vi "test game logic.vi"() -> ()   [LabVIEW 2024]
uses:
  state machine variables.ctl
  state machine states.ctl
  state machine controller.ctl
panel:
  out "Sequence":dbl[](array[numeric])
  in  "Button 4":bool
  in  "Button3":bool
  in  "Button 2":bool
  in  "Button 1":bool
  in  "Round":dbl
  in  "Score":dbl
  in  "stop":bool
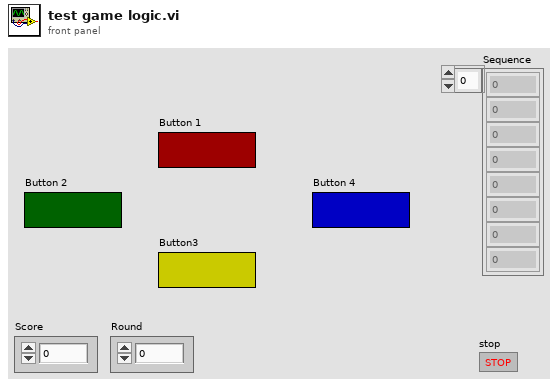
[diagram p1: front panel]
types:
  T1 = typedef "state machine states.ctl" = enum16{"Initialize", "update display", "Show sequence", "User response", "update data", ""}
  T2 = typedef "state machine variables.ctl" = cluster{"Sequence":dbl[], "Score":dbl, "Round":dbl}
  T3 = typedef "VI Communication.ctl" = cluster{"Queue":refnum<queue>, "Path":path, "Score":dbl, "Level":dbl}
  T4 = typedef "state machine controller.ctl" = cluster{"State Machine State":string, "Difficulty":dbl, "Login User Name":string, "Login User Passwd":string}
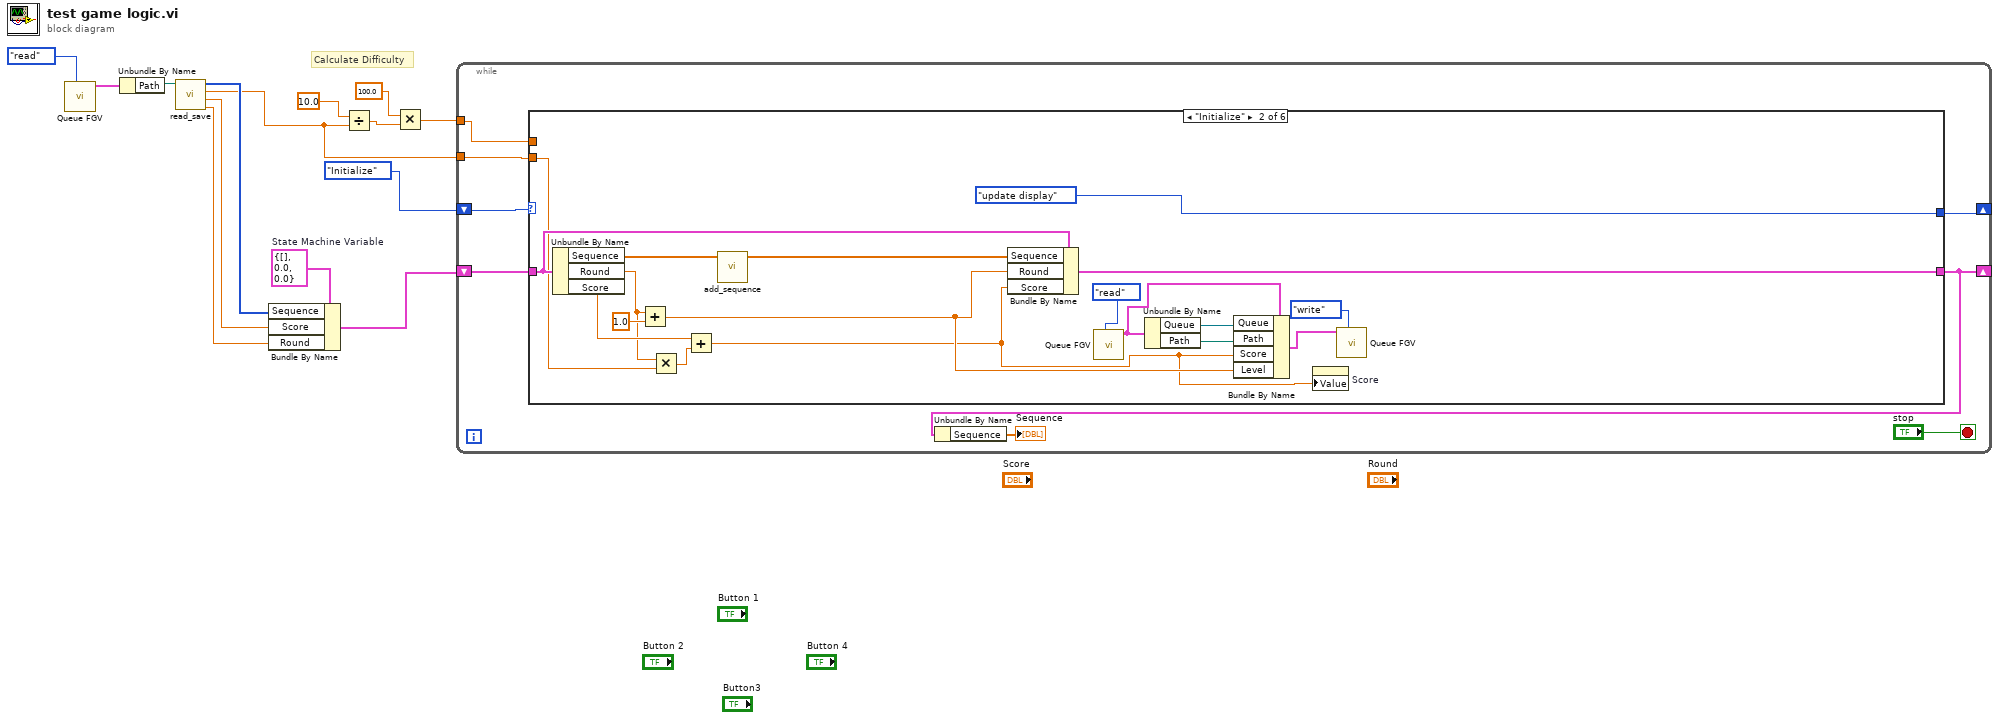
[diagram p0: block diagram]
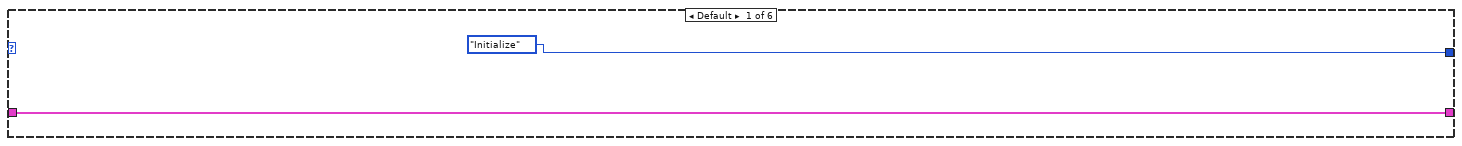
[diagram p2: hidden frame]
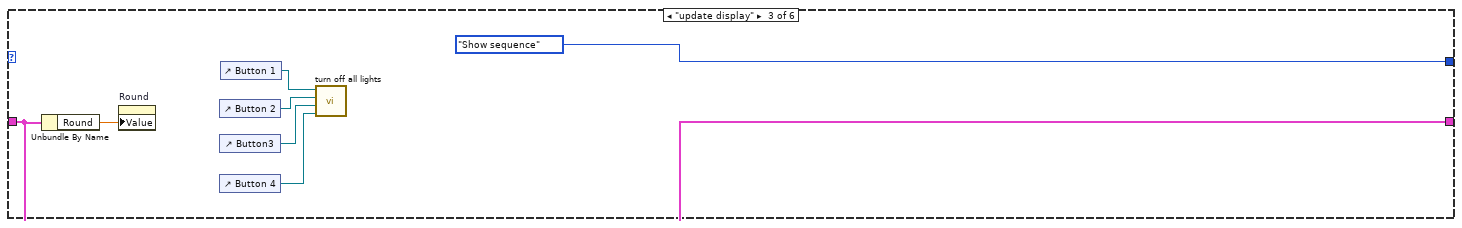
[diagram p3: hidden frame]
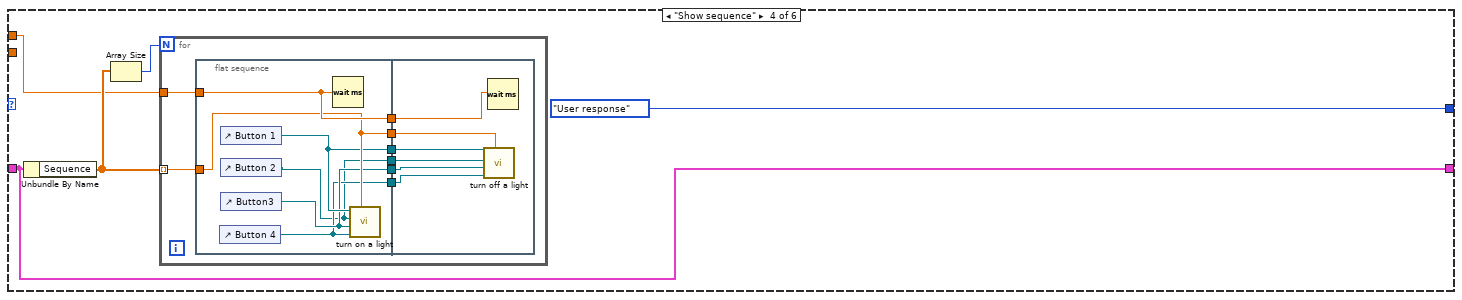
[diagram p4: hidden frame]
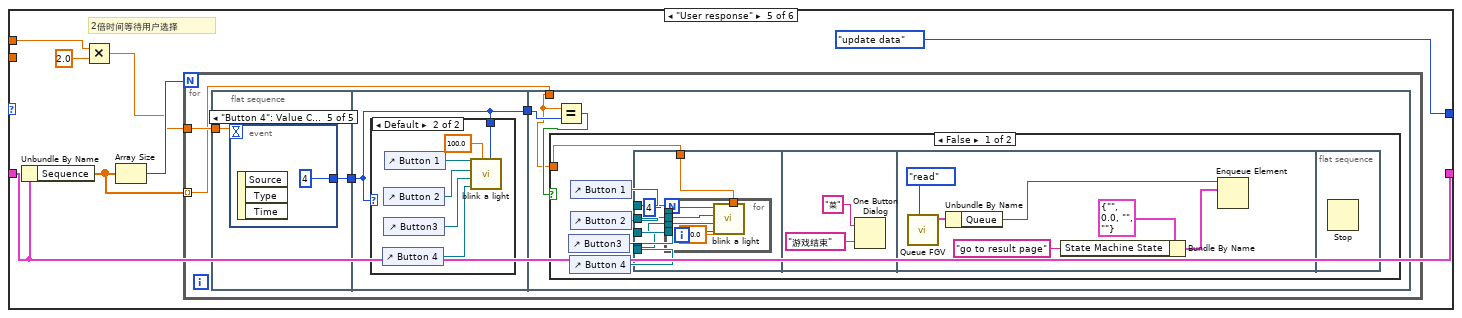
[diagram p5: hidden frame]
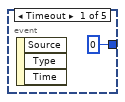
[diagram p6: hidden frame]
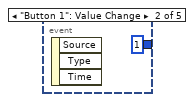
[diagram p7: hidden frame]
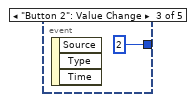
[diagram p8: hidden frame]
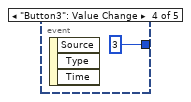
[diagram p9: hidden frame]
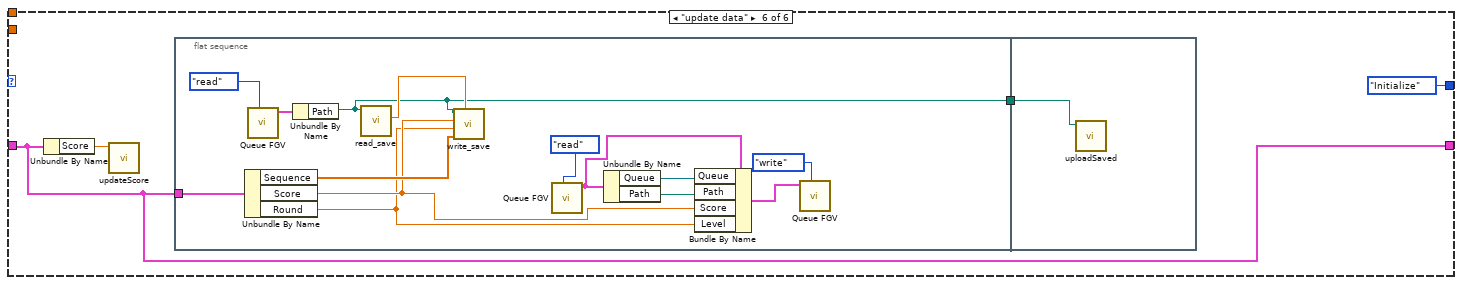
[diagram p12: hidden frame]
diagram:
  w6 = T2 {"Sequence"=[], "Score"=0.0, "Round"=0.0}  # State Machine Variable
  # "Calculate Difficulty"
  n1 = call "Queue FGV.vi"("Enum"=enum16{"read", "write"}."read") -> ("VI Communication Out"=w8:T3)  [unwired: 10 in]
  n2 = Unbundle By Name(w8) -> ("Path"=w7:path)
  n3 = call "read_save.vi"("save file path"=w7) -> ("Level"=w4:dbl, "Score"=w3:dbl, "Difficulty"=w1:dbl, "Sequence Array"=w2:i32[])  [unwired: 6 in, 1 out]
  n4 = Bundle By Name(cluster=w6, "Sequence"=w2, "Score"=w3, "Round"=w4) -> (w5:T2)
  n5 = Divide(x=10.0, y=w1) -> (x/y=w12:dbl)
  n6 = Multiply(x=100.0, y=w12) -> (x*y=w11:dbl)
  n7 = while {
    shift-right: [w16] -> _
    shift-left: w5 -> [w22]
    shift-right: [w19] -> _
    shift-left: state_machine_states."Initialize" -> [w20]
    tunnel: w11 -> [w18]
    tunnel: w1 -> [w15]
    stop <- "stop" stop-if-true
    n8 = case shown="\"Initialize\"" w20 {
      tunnel: w22 -> [w24 w41 w49 w50 w75 w128]
      tunnel: [w24 w40 w49 w50 w75 w128] -> w16
      tunnel: [state_machine_states."Initialize" ("Enum") state_machine_states."update display" ("Enum") state_machine_states."Show sequence" ("Enum") state_machine_states."User response" ("Enum") state_machine_states."update data" ("Enum") state_machine_states."Initialize" ("Enum")] -> w19
      tunnel: w18 -> [_ _ _ w52 w77 _]
      tunnel: w15 -> [_ w33 _ _ _ _]
      frame Default {
      }
      frame "Initialize" {
        n9 = Unbundle By Name(w41) -> ("Sequence"=w42:dbl[], "Round"=w34:dbl, "Score"=w35:dbl)
        n10 = Add(x=w34, y=1.0) -> (x+y=w27:dbl)
        n11 = Multiply(x=w34, y=w33) -> (x*y=w36:dbl)
        n12 = Add(x=w35, y=w36) -> (x+y=w26:dbl)
        n13 = call "add_sequence.vi"("sequence in"=w42) -> ("sequence out"=w39:dbl[])  [unwired: 9 in, 1 out]
        n14 = Bundle By Name(cluster=w41, "Sequence"=w39, "Round"=w27, "Score"=w26) -> (w40:T2)
        n15 = call "Queue FGV.vi"("Enum"=enum16{"read", "write"}."read") -> ("VI Communication Out"=w31:T3)  [unwired: 10 in]
        n16 = Unbundle By Name(w31) -> ("Queue"=w29:refnum<queue>, "Path"=w28:path)
        n17 = Bundle By Name(cluster=w31, "Queue"=w29, "Path"=w28, "Score"=w26, "Level"=w27) -> (w25:T3)
        n18 = property on="Score" class="DigNum (strict)"("Value"=w26) -> ()  [unwired: 2 in, 2 out]
        n19 = call "Queue FGV.vi"("Enum"=enum16{"read", "write"}."write", "VI Communication In"=w25) -> ()  [unwired: 9 in, 1 out]
      }
      frame "update display" {
        n20 = Unbundle By Name(w49) -> ("Round"=w48:dbl)
        n21 = property on="Round" class="DigNum (strict)"("Value"=w48) -> ()  [unwired: 2 in, 2 out]
        n22 = control-ref of="Button 2"() -> (w45:refnum<vi>)
        n23 = control-ref of="Button3"() -> (w44:refnum<vi>)
        n24 = control-ref of="Button 4"() -> (w43:refnum<vi>)
        n25 = control-ref of="Button 1"() -> (w46:refnum<vi>)
        n26 = call "turn off all lights.vi"("Button 4"=w43, "Button 3"=w44, "Button 2"=w45, "Button 1"=w46) -> ()  [unwired: 7 in, 1 out]
      }
      frame "Show sequence" {
        n27 = Unbundle By Name(w50) -> ("Sequence"=w53:dbl[])
        n28 = Array Size(array=w53) -> (size(s)=w54:i32)
        n29 = for {
          N: w54 -> [_]
          tunnel: w53 -> [w62] mode=indexing
          tunnel: w52 -> [w61]
          n30 = flat-sequence {
            tunnel: w62 -> [w67]
            tunnel: w61 -> [w68]
            tunnel: [w68] -> w60
            tunnel: [w67] -> w59
            tunnel: [w66] -> w58
            tunnel: [w65] -> w57
            tunnel: [w64] -> w56
            tunnel: [w63] -> w55
            tunnel: w60 -> [w74]
            tunnel: w59 -> [w73]
            tunnel: w58 -> [w72]
            tunnel: w57 -> [w71]
            tunnel: w56 -> [w70]
            tunnel: w55 -> [w69]
            frame #0 {
              n31 = control-ref of="Button 4"() -> (w64:refnum<vi>)
              n32 = control-ref of="Button 1"() -> (w66:refnum<vi>)
              n33 = control-ref of="Button 2"() -> (w63:refnum<vi>)
              n34 = control-ref of="Button3"() -> (w65:refnum<vi>)
              n35 = Wait (ms)(milliseconds to wait=w68) -> ()  [unwired: 1 out]
              n36 = call "turn on a light.vi"("Which Button?"=w67, "Button 4"=w64, "Button 3"=w65, "Button 2"=w63, "Button 1"=w66) -> ()  [unwired: 6 in, 1 out]
            }
            frame #1 {
              n37 = call "turn off a light.vi"("Which Button?"=w73, "Button 4"=w70, "Button 3"=w71, "Button 2"=w69, "Button 1"=w72) -> ()  [unwired: 6 in, 1 out]
              n38 = Wait (ms)(milliseconds to wait=w74) -> ()  [unwired: 1 out]
            }
          }
        }
      }
      frame "User response" {
        # "2倍时间等待用户选择"
        n39 = Unbundle By Name(w75) -> ("Sequence"=w79:dbl[])
        n40 = Multiply(x=w77, y=2.0) -> (x*y=w78:dbl)
        n41 = Array Size(array=w79) -> (size(s)=w80:i32)
        n42 = for {
          N: w80 -> [_]
          tunnel: w79 -> [w83] mode=indexing
          tunnel: w78 -> [w85]
          n43 = flat-sequence {
            tunnel: w85 -> [w87]
            tunnel: [w86] -> w84
            tunnel: w84 -> [w93]
            tunnel: [w93] -> w82
            tunnel: w83 -> [w100]
            tunnel: w82 -> [w102]
            frame #0 {
              n44 = event shown="[4] \"Button 4\": Value Change" {
                selector: _ -> [_ _ _ _ _]
                dyn-events: _ -> [_ _ _ _ _]
                timeout: w87 -> [_ _ _ _ _]
                tunnel: [u32 0 1 2 3 u32 4] -> w86
                event Timeout {
                  n45 = event-data() -> ()  [unwired: 1 in, 3 out]
                }
                event "Button 1": Value Change {
                  n46 = event-data() -> ()  [unwired: 1 in, 3 out]
                }
                event "Button 2": Value Change {
                  n47 = event-data() -> ()  [unwired: 1 in, 3 out]
                }
                event "Button3": Value Change {
                  n48 = event-data() -> ()  [unwired: 1 in, 3 out]
                }
                event "Button 4": Value Change {
                  n49 = event-data() -> ()  [unwired: 1 in, 3 out]
                }
              }
            }
            frame #1 {
              n50 = case shown="Default" w93 {
                tunnel: w93 -> [_ w99]
                frame 0 {
                }
                frame Default {
                  n51 = control-ref of="Button 4"() -> (w95:refnum<vi>)
                  n52 = control-ref of="Button 2"() -> (w97:refnum<vi>)
                  n53 = control-ref of="Button3"() -> (w96:refnum<vi>)
                  n54 = control-ref of="Button 1"() -> (w98:refnum<vi>)
                  n55 = call "blink a light.vi"("Whcih Button?"=w99, "Blink Time"=100.0, "Button 4"=w95, "Button 3"=w96, "Button 2"=w97, "Button 1"=w98) -> ()  [unwired: 5 in, 1 out]
                }
              }
            }
            frame #2 {
              n56 = Equal?(x=w100, y=w102) -> (x = y?=w101:bool)
              n57 = case shown="False" w101 {
                tunnel: w100 -> [w107 _]
                frame False {
                  n58 = control-ref of="Button3"() -> (w104:refnum<vi>)
                  n59 = control-ref of="Button 4"() -> (w103:refnum<vi>)
                  n60 = control-ref of="Button 1"() -> (w106:refnum<vi>)
                  n61 = control-ref of="Button 2"() -> (w105:refnum<vi>)
                  n62 = flat-sequence {
                    tunnel: w107 -> [w113]
                    tunnel: w106 -> [w110]
                    tunnel: w105 -> [w109]
                    tunnel: w104 -> [w111]
                    tunnel: [w112] -> _
                    tunnel: w103 -> [w112]
                    frame #0 {
                      n63 = for {
                        N: 4 -> [_]
                        tunnel: w113 -> [w119]
                        tunnel: w112 -> [w118]
                        tunnel: w111 -> [w117]
                        tunnel: w110 -> [w116]
                        tunnel: w109 -> [w115]
                        n64 = call "blink a light.vi"("Whcih Button?"=w119, "Blink Time"=200.0, "Button 4"=w118, "Button 3"=w117, "Button 2"=w115, "Button 1"=w116) -> ()  [unwired: 5 in, 1 out]
                      }
                    }
                    frame #1 {
                      n65 = One Button Dialog(message="菜", button name ("OK")="游戏结束") -> ()  [unwired: 1 out]
                    }
                    frame #2 {
                      n66 = call "Queue FGV.vi"("Enum"=enum16{"read", "write"}."read") -> ("VI Communication Out"=w122:T3)  [unwired: 10 in]
                      n67 = Unbundle By Name(w122) -> ("Queue"=w126:refnum<queue>)
                      n68 = Bundle By Name(cluster=T4 {"State Machine State"="", "Difficulty"=0.0, "Login User Name"="", "Login User Passwd"=""} ("Cluster"), "State Machine State"="go to result page") -> (w123:T4)
                      n69 = Enqueue Element(queue=w126, element=w123) -> ()  [unwired: 2 in, 3 out]
                    }
                    frame #3 {
                      n70 = Stop() -> ()  [unwired: 1 in]
                    }
                  }
                }
                frame True {
                }
              }
            }
          }
        }
      }
      frame "update data" {
        n71 = Unbundle By Name(w128) -> ("Score"=w131:dbl)
        n72 = call "updateScore.vi"("New Score"=w131) -> ()  [unwired: 10 in, 1 out]
        n73 = flat-sequence {
          tunnel: w128 -> [w143]
          tunnel: [w140] -> w130
          tunnel: w130 -> [w146]
          frame #0 {
            n74 = Unbundle By Name(w143) -> ("Sequence"=w141:dbl[], "Score"=w133:dbl, "Round"=w132:dbl)
            n75 = call "Queue FGV.vi"("Enum"=enum16{"read", "write"}."read") -> ("VI Communication Out"=w144:T3)  [unwired: 10 in]
            n76 = Unbundle By Name(w144) -> ("Path"=w140:path)
            n77 = call "read_save.vi"("save file path"=w140) -> ("Difficulty"=w142:dbl)  [unwired: 6 in, 4 out]
            n78 = call "write_save.vi"("Difficulty"=w142, "Sequence"=w141, "Level"=w132, "Score"=w133, "save file path"=w140) -> ()  [unwired: 6 in, 1 out]
            n79 = call "Queue FGV.vi"("Enum"=enum16{"read", "write"}."read") -> ("VI Communication Out"=w138:T3)  [unwired: 10 in]
            n80 = Unbundle By Name(w138) -> ("Queue"=w135:refnum<queue>, "Path"=w134:path)
            n81 = Bundle By Name(cluster=w138, "Queue"=w135, "Path"=w134, "Score"=w133, "Level"=w132) -> (w137:T3)
            n82 = call "Queue FGV.vi"("Enum"=enum16{"read", "write"}."write", "VI Communication In"=w137) -> ()  [unwired: 9 in, 1 out]
          }
          frame #1 {
            n83 = call "uploadSaved.vi"("Path"=w146) -> ()  [unwired: 10 in, 1 out]
          }
        }
      }
    }
    n84 = Unbundle By Name(w16) -> ("Sequence"=→"Sequence":dbl[])
  }
